vi "DQtoABC_src.vi"(0 "direct":sgl format="%#_30g", 5 "quadrature":sgl format="%#_30g", 7 "theta":sgl) -> (4 "A":sgl format="%#_32g", 6 "B":sgl, 8 "C":sgl, 10 "alpha":sgl format="%#_30g", 15 "beta":sgl format="%#_30g")   [LabVIEW 2015]
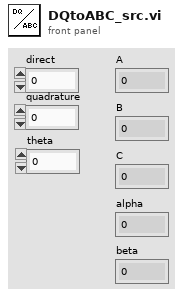
[diagram p1: front panel]
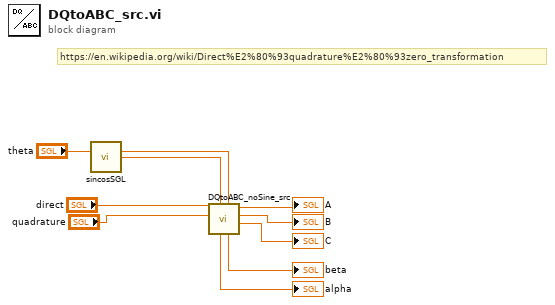
[diagram p0: block diagram]
diagram:
  # "https://en.wikipedia.org/wiki/Direct%E2%80%93quadrature%E2%80%93zero_transformation"
  n1 = call "sincosSGL.vi"("x"="theta") -> ("sinx"=w6:sgl, "cosx"=w7:sgl)  [unwired: 13 in]
  n2 = call "DQtoABC_noSine_src.vi"("sinx"=w6, "cosx"=w7, "quadrature"="quadrature", "direct"="direct") -> ("C"=→"C":sgl, "B"=→"B":sgl, "A"=→"A":sgl, "beta"=→"beta":sgl, "alpha"=→"alpha":sgl)  [unwired: 3 in]
